vi "displayDetailedState.vi"(10 "viewThisComponent":refnum<class "ViewThisComponent.lvclass">) -> ()   [LabVIEW 2016, in "calibrationSpectrometerViewElements.lvlib"]
doc: "Displays information about the detailed state."
uses:
  calibrationSpectrometerViewElements.lvlib
  ViewThisComponent/ViewThisComponent.lvclass
  home/harini/tcs/ts_sedspectrometer/ComponentTemplateCore/ComponentModel/ComponentModel/View/View.lvclass
  ComponentTemplateCore/ComponentModel/ComponentModel/View/View.lvclass
panel:
  out "SED:":string caption="EXA:"
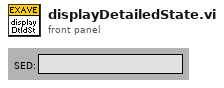
[diagram p1: front panel]
types:
  T1 = typedef "TypedefsDataEvents.lvlib/PubDataEvents.ctl" = cluster{"AppliedSettingsMatchStart":refnum<user-event>, "SettingVersions":refnum<user-event>, "SummaryState":refnum<user-event>, "RejectedCommand":refnum<user-event>, "DetailedState":refnum<user-event>, "ErrorCode":refnum<user-event>, "Heartbeat":refnum<user-event>, "LoopTime_ms":refnum<user-event>, "LoopTimeOutOfRange":refnum<user-event>, "Timestamp":refnum<user-event>, "TimeOut":refnum<user-event>, "MeasuredSpectrum":refnum<user-event>}
  T2 = enum16{"", "DisabledState", "EnabledState", "FaultState", "OfflineState", "StandbyState"}
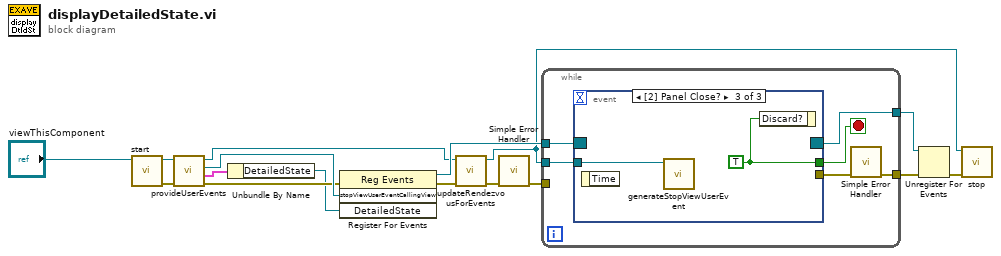
[diagram p0: block diagram]
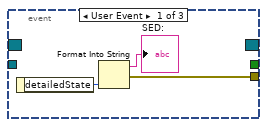
[diagram p2: hidden frame]
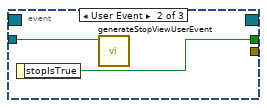
[diagram p3: hidden frame]
diagram:
  n1 = call-dynamic "start.vi"("View in"="viewThisComponent") -> ("error out"=w12:errorcluster, "View out"=w13:refnum<class "ViewThisComponent.lvclass">)  [unwired: 9 in]
  n2 = call "provideUserEvents.vi"("error in (no error)"=w12, "ViewThisComponent in"=w13) -> ("error out"=w11:errorcluster, "pubDataEvents"=w14:T1, "stopViewUserEventCallingView"=w15:refnum<user-event>, "ViewThisComponent out"=w2:refnum<class "ViewThisComponent.lvclass">)  [unwired: 6 in]
  n3 = Unbundle By Name(w14) -> ("DetailedState"=w6:refnum<user-event>)
  n4 = register-events(error in=w11, w15, w6) -> (reference out=w10:refnum<event-registration>, error out=w4:errorcluster)  [unwired: 1 in]
  n5 = call "updateRendezvousForEvents.vi"("error in (no error)"=w4, "View in"=w2) -> ("error out"=w3:errorcluster, "View out"=w1:refnum<class "ViewThisComponent.lvclass">)  [unwired: 8 in]
  n6 = call <vilib>:"Simple Error Handler.vi"("error in (no error)"=w3) -> ("error out"=w5:errorcluster)  [unwired: 4 in, 4 out]
  n7 = while {
    tunnel: w10 -> [w22]
    tunnel: [w20] -> w9
    tunnel: w1 -> [w19]
    tunnel: [w17] -> w7
    tunnel: w5 -> [_]
    stop <- w18 stop-if-true
    n8 = event shown="[2] Panel Close?" {
      selector: w22 -> [_ _ _]
      dyn-events: [_ _ _] -> w17
      timeout: _ -> [_ _ _]
      tunnel: [w25 _ _] -> w21
      tunnel: w19 -> [_ w26 w29]
      tunnel: [_ w27 w28] -> w18
      event User Event {
        n9 = event-data() -> ("detailedState"=w24:T2)  [unwired: 1 in]
        n10 = Format Into String(w24) -> (resulting string=→"SED:":string, error out=w25:errorcluster)  [unwired: 3 in]
      }
      event User Event {
        n11 = event-data() -> ("stopIsTrue"=w27:bool)  [unwired: 1 in]
        n12 = call "generateStopViewUserEvent.vi"("View in"=w26) -> ()  [unwired: 9 in, 2 out]
      }
      event Panel Close? {
        w28 = TRUE ("Discard?")
        n13 = event-data() -> ()  [unwired: 1 in, 1 out]
        n14 = call "generateStopViewUserEvent.vi"("View in"=w29) -> ()  [unwired: 9 in, 2 out]
        n15 = event-data("Discard?"=w28) -> ()  [unwired: 1 in, 1 out]
      }
    }
    n16 = call <vilib>:"Simple Error Handler.vi"("error in (no error)"=w21) -> ("error out"=w20:errorcluster)  [unwired: 4 in, 4 out]
  }
  n17 = Unregister For Events(event registration refnum=w7, error in=w9) -> (error out=w8:errorcluster)
  n18 = call-dynamic "stop.vi"("error in (no error)"=w8, "View in"=w1) -> ()  [unwired: 8 in, 2 out]
